vi "Parse Error XML.vi"(9 "Code Tag Value":string, 10 "Error XML":string) -> (0 "Unknown Error":bool, 1 "Error Description Override":string, 2 "Error Code":i32, 3 "Warning":bool)   [LabVIEW 2015, in "NI_Azure_Blob.lvlib"]
uses:
  NI_Azure_Blob.lvlib
  Core/NI_Azure_Core.lvlib
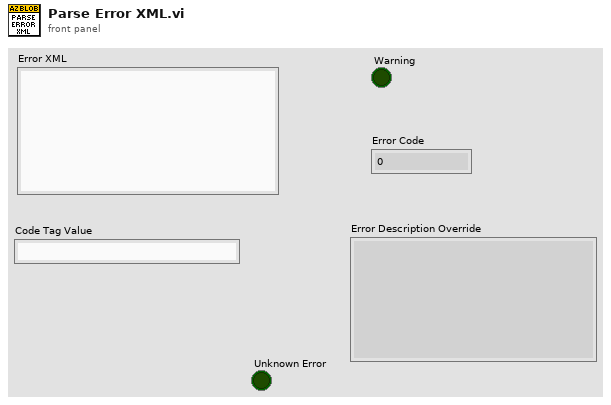
[diagram p1: front panel]
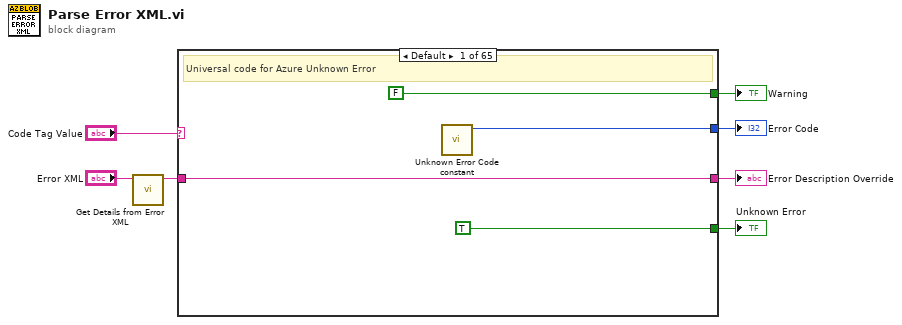
[diagram p0: block diagram]
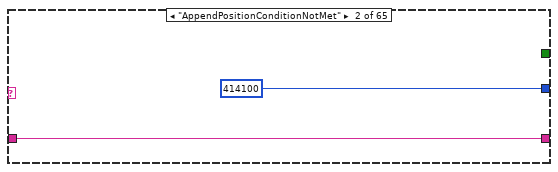
[diagram p2: hidden frame]
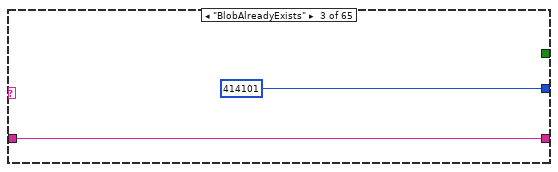
[diagram p3: hidden frame]
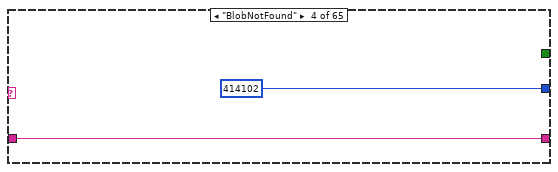
[diagram p4: hidden frame]
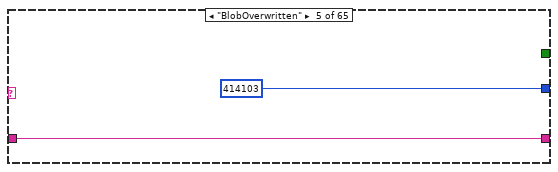
[diagram p5: hidden frame]
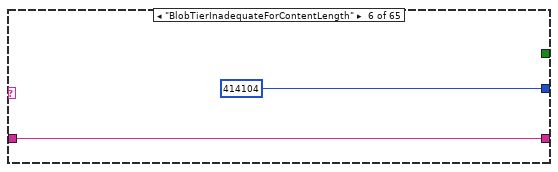
[diagram p6: hidden frame]
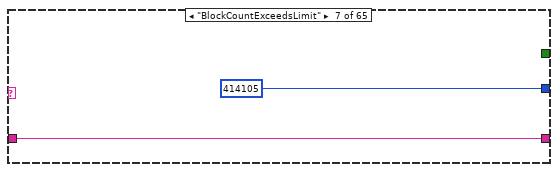
[diagram p7: hidden frame]
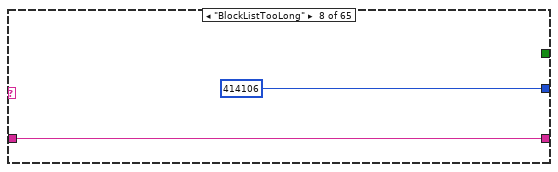
[diagram p8: hidden frame]
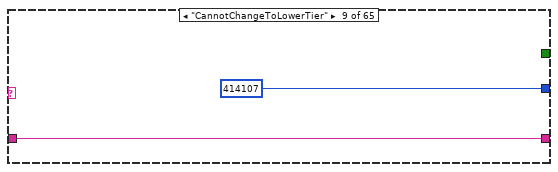
[diagram p9: hidden frame]
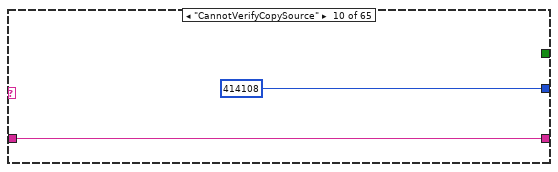
[diagram p10: hidden frame]
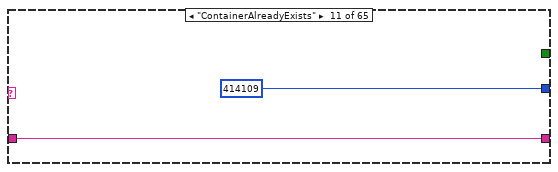
[diagram p11: hidden frame]
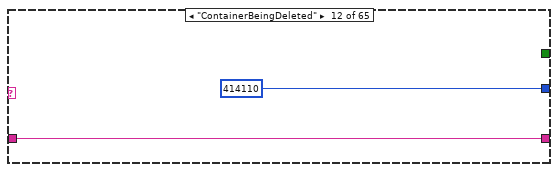
[diagram p12: hidden frame]
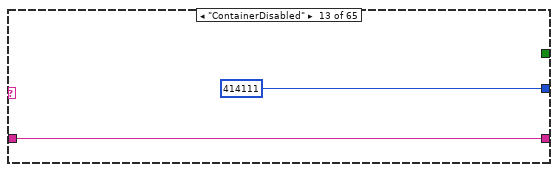
[diagram p13: hidden frame]
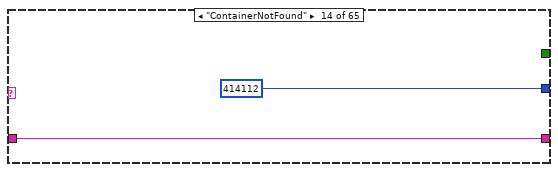
[diagram p14: hidden frame]
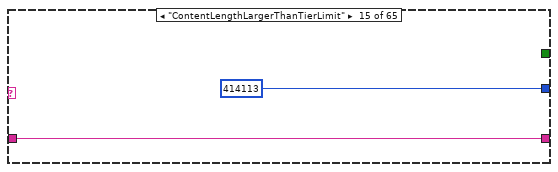
[diagram p15: hidden frame]
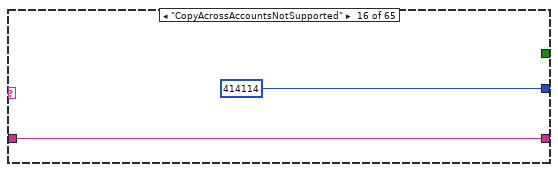
[diagram p16: hidden frame]
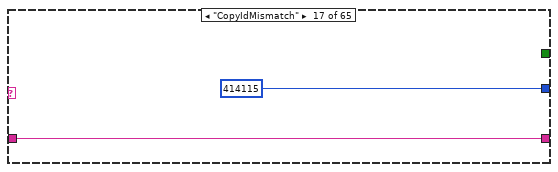
[diagram p17: hidden frame]
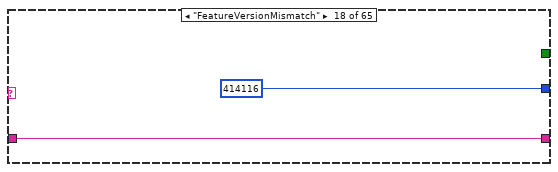
[diagram p18: hidden frame]
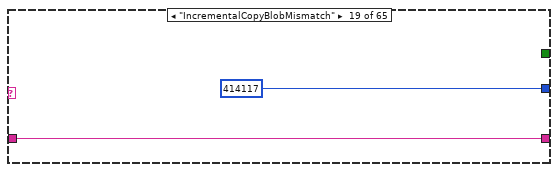
[diagram p19: hidden frame]
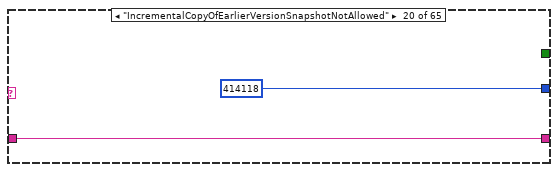
[diagram p20: hidden frame]
diagram:
  n1 = call "Get Details from Error XML.vi"("Error XML"="Error XML") -> ("Details"=w1:string)  [unwired: 10 in]
  n2 = case shown="Default" "Code Tag Value" {
    tunnel: [w10 414100 414101 414102 414103 414104 414105 414106 414107 414108 414109 414110 414111 414112 414113 414114 414115 414116 414117 414118 414119 414120 414121 414122 414123 414124 414125 414126 414127 414128 414129 414130 414131 414132 414133 414134 414135 414136 414137 414138 414139 414140 414141 414142 414143 414144 414145 414146 414147 414148 414149 414150 414151 414152 414153 414154 414155 414156 414157 414158 414159 414160 414161 414162 414163] -> w5
    tunnel: [FALSE _ _ _ _ _ _ _ _ _ _ _ _ _ _ _ _ _ _ _ _ _ _ _ _ _ _ _ _ _ _ _ _ _ _ _ _ _ _ _ _ _ _ _ _ _ _ _ _ _ _ _ _ _ _ _ _ _ _ _ _ _ _ _ _] -> w6
    tunnel: w1 -> [w9 w12 w14 w16 w18 w20 w22 w24 w26 w28 w30 w32 w34 w36 w38 w40 w42 w44 w46 w48 w50 w52 w54 w56 w58 w60 w62 w64 w66 w68 w70 w72 w74 w76 w78 w80 w82 w84 w86 w88 w90 w92 w94 w96 w98 w100 w102 w104 w106 w108 w110 w112 w114 w116 w118 w120 w122 w124 w126 w128 w130 w132 w134 w136 w138]
    tunnel: [w9 w12 w14 w16 w18 w20 w22 w24 w26 w28 w30 w32 w34 w36 w38 w40 w42 w44 w46 w48 w50 w52 w54 w56 w58 w60 w62 w64 w66 w68 w70 w72 w74 w76 w78 w80 w82 w84 w86 w88 w90 w92 w94 w96 w98 w100 w102 w104 w106 w108 w110 w112 w114 w116 w118 w120 w122 w124 w126 w128 w130 w132 w134 w136 w138] -> w4
    tunnel: [TRUE _ _ _ _ _ _ _ _ _ _ _ _ _ _ _ _ _ _ _ _ _ _ _ _ _ _ _ _ _ _ _ _ _ _ _ _ _ _ _ _ _ _ _ _ _ _ _ _ _ _ _ _ _ _ _ _ _ _ _ _ _ _ _ _] -> w3
    frame Default {
      # "Universal code for Azure Unknown Error"
      n3 = call "Unknown Error Code constant.vi"() -> ("Azure Unknown Error Code value"=w10:i32)  [unwired: 11 in]
    }
    frame "AppendPositionConditionNotMet" {
    }
    frame "BlobAlreadyExists" {
    }
    frame "BlobNotFound" {
    }
    frame "BlobOverwritten" {
    }
    frame "BlobTierInadequateForContentLength" {
    }
    frame "BlockCountExceedsLimit" {
    }
    frame "BlockListTooLong" {
    }
    frame "CannotChangeToLowerTier" {
    }
    frame "CannotVerifyCopySource" {
    }
    frame "ContainerAlreadyExists" {
    }
    frame "ContainerBeingDeleted" {
    }
    frame "ContainerDisabled" {
    }
    frame "ContainerNotFound" {
    }
    frame "ContentLengthLargerThanTierLimit" {
    }
    frame "CopyAcrossAccountsNotSupported" {
    }
    frame "CopyIdMismatch" {
    }
    frame "FeatureVersionMismatch" {
    }
    frame "IncrementalCopyBlobMismatch" {
    }
    frame "IncrementalCopyOfEarlierVersionSnapshotNotAllowed" {
    }
    frame "IncrementalCopySourceMustBeSnapshot" {
    }
    frame "InfiniteLeaseDurationRequired" {
    }
    frame "InvalidBlobOrBlock" {
    }
    frame "InvalidBlobTier" {
    }
    frame "InvalidBlobType" {
    }
    frame "InvalidBlockId" {
    }
    frame "InvalidBlockList" {
    }
    frame "InvalidOperation" {
    }
    frame "InvalidPageRange" {
    }
    frame "InvalidSourceBlobType" {
    }
    frame "InvalidSourceBlobUrl" {
    }
    frame "InvalidVersionForPageBlobOperation" {
    }
    frame "LeaseAlreadyPresent" {
    }
    frame "LeaseAlreadyBroken" {
    }
    frame "LeaseIdMismatchWithBlobOperation" {
    }
    frame "LeaseIdMismatchWithContainerOperation" {
    }
    frame "LeaseIdMismatchWithLeaseOperation" {
    }
    frame "LeaseIdMissing" {
    }
    frame "LeaseIsBreakingAndCannotBeAcquired" {
    }
    frame "LeaseIsBreakingAndCannotBeChanged" {
    }
    frame "LeaseIsBrokenAndCannotBeRenewed" {
    }
    frame "LeaseLost" {
    }
    frame "LeaseNotPresentWithBlobOperation" {
    }
    frame "LeaseNotPresentWithContainerOperation" {
    }
    frame "LeaseNotPresentWithLeaseOperation" {
    }
    frame "MaxBlobSizeConditionNotMet" {
    }
    frame "NoPendingCopyOperation" {
    }
    frame "OperationNotAllowedOnIncrementalCopyBlob" {
    }
    frame "PendingCopyOperation" {
    }
    frame "PreviousSnapshotCannotBeNewer" {
    }
    frame "PreviousSnapshotNotFound" {
    }
    frame "PreviousSnapshotOperationNotSupported" {
    }
    frame "SequenceNumberConditionNotMet" {
    }
    frame "SequenceNumberIncrementTooLarge" {
    }
    frame "SnapshotCountExceeded" {
    }
    frame "SnaphotOperationRateExceeded" {
    }
    frame "SnapshotsPresent" {
    }
    frame "SourceConditionNotMet" {
    }
    frame "SystemInUse" {
    }
    frame "TargetConditionNotMet" {
    }
    frame "UnauthorizedBlobOverwrite" {
    }
    frame "UnsupportedHeader" {
    }
    frame "BlobBeingRehydrated" {
    }
    frame "BlobArchived" {
    }
    frame "BlobNotArchived" {
    }
  }
  "Error Description Override" <- w4
  "Warning" <- w6
  "Error Code" <- w5
  "Unknown Error" <- w3
